vi "WPI_Power Get PDP Currents.vi"(0 "Power Distribution Panel (0)":u8, 5 "PDP Channel":i32, 7 "Tare Currents?":bool, 11 "error in":errorcluster) -> (6 "current (A)":dbl, 8 "all currents (A)":dbl[](array[numeric]), 15 "error out":errorcluster)   [LabVIEW 2017]
doc: "Returns the currents of the Power Distribution Panel (PDP) channels."
uses:
  <vilib>/Rock Robotics/WPI/CAN/PDP/WPI_CAN_PDPGlobalOps.ctl
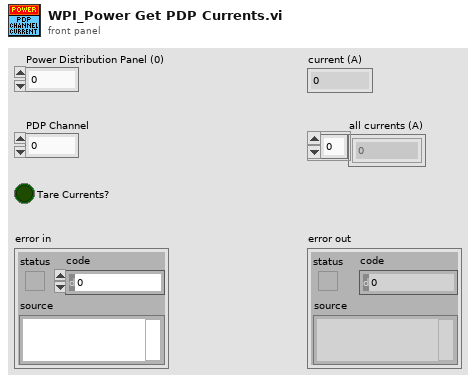
[diagram p1: front panel]
types:
  T1 = typedef "WPI_CAN_PDPGlobalOps.ctl" = enum16{"Write After Receive 0-5", "Write After Receive 6-11", "Write After Receive 12-15", "Write After Receive Energy", "Get All", "Get Commands", "Write Clear Sticky Faults Command", "Write Reset Energy Command", "Write Tare Currents Command", "Write Error", "Write After Receive Faults"}
  T2 = typedef "WPI_CAN_PDPGetAll.ctl" = cluster{"Channel Currents":dbl[], "Battery Voltage":dbl, "Temperature (degrees C)":dbl, "Internal Battery R (Ohms)":dbl, "Energy (J)":dbl, "Power (W)":dbl, "Total Current (A)":dbl, "CAN Error":errorcluster, "Current Faults":bool[], "Battery Voltage Fault":bool, "Temperature Fault":bool, "Hardware Fault":bool}
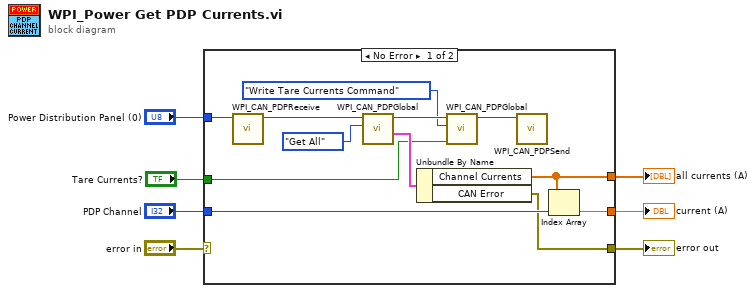
[diagram p0: block diagram]
diagram:
  n1 = case shown="No Error" "error in" {
    selector: "error in" -> [_ w20]
    tunnel: [w8 w20] -> w6
    tunnel: "Power Distribution Panel (0)" -> [w17 _]
    tunnel: [w15 _] -> w4
    tunnel: [w14 _] -> w3
    tunnel: "PDP Channel" -> [w13 _]
    tunnel: "Tare Currents?" -> [w10 _]
    frame No Error {
      n2 = call <vilib>:"WPI_CAN_PDPReceive.vi"("Power Distribution Panel (0)"=w17) -> ("Power Distribution Panel Out"=w18:u8)  [unwired: 10 in]
      n3 = call <vilib>:"WPI_CAN_PDPGlobal.vi"("Operation"=WPI_CAN_PDPGlobalOps."Get All", "Power Distribution Panel (0)"=w18) -> ("Get All"=w19:T2, "Power Distribution Panel Out"=w12:u8)  [unwired: 7 in, 1 out]
      n4 = Unbundle By Name(w19) -> ("Channel Currents"=w15:dbl[], "CAN Error"=w8:errorcluster)
      n5 = call <vilib>:"WPI_CAN_PDPGlobal.vi"("Command"=w10, "Operation"=WPI_CAN_PDPGlobalOps."Write Tare Currents Command", "Power Distribution Panel (0)"=w12) -> ("Power Distribution Panel Out"=w9:u8)  [unwired: 6 in, 2 out]
      n6 = call <vilib>:"WPI_CAN_PDPSend.vi"("Power Distribution Panel (0)"=w9) -> ()  [unwired: 10 in, 1 out]
      n7 = Index Array(array=w15, index=w13) -> (element=w14:dbl)
    }
    frame Error {
    }
  }
  "error out" <- w6
  "current (A)" <- w3
  "all currents (A)" <- w4
